vi "String Operations.vi"() -> ()   [LabVIEW 2020]
panel:
  out "offset past replacement":i32
  out "number of replacements":i32
  out "result string 2":string
  in  "Replace str":string
  in  "input str":string="I'm trying to remember something but I couldn't. It's something important , still I forgot. "
  in  "search str":string
  out "result string":string
  out "replaced substring":string
  out "substring":string
  out "len t str":i32
  out "len str3":i32
  out "trimmed string":string
  in  "Str 3":string
  out "concatenated string":string
  in  "Str 2":string
  in  "Str":string
  # "STRING OPERATIONS"
  # "+"
  # "="
  # "t str (2-5)"
  # "string =str3 and substring = str2"
  # "Search and Replace string function"
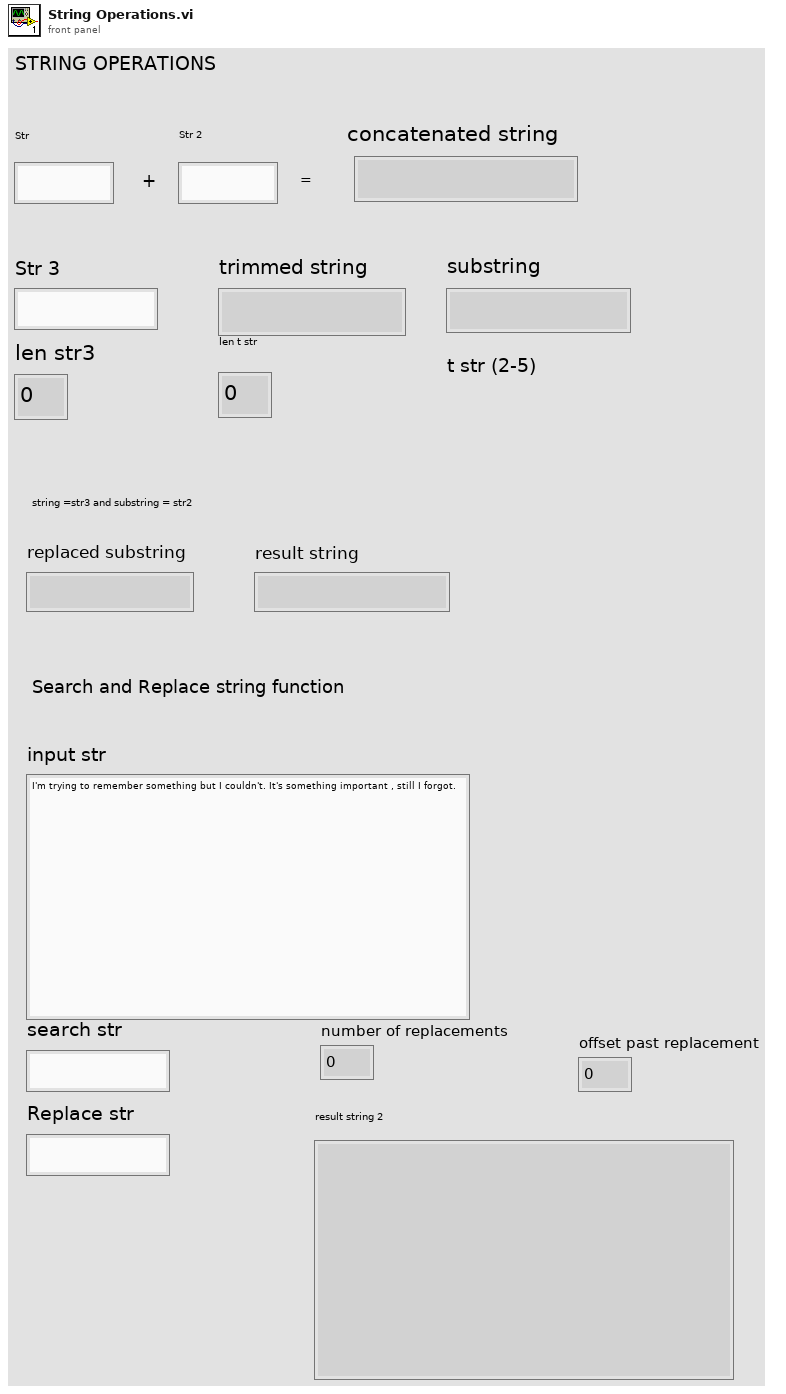
[diagram p1: front panel]
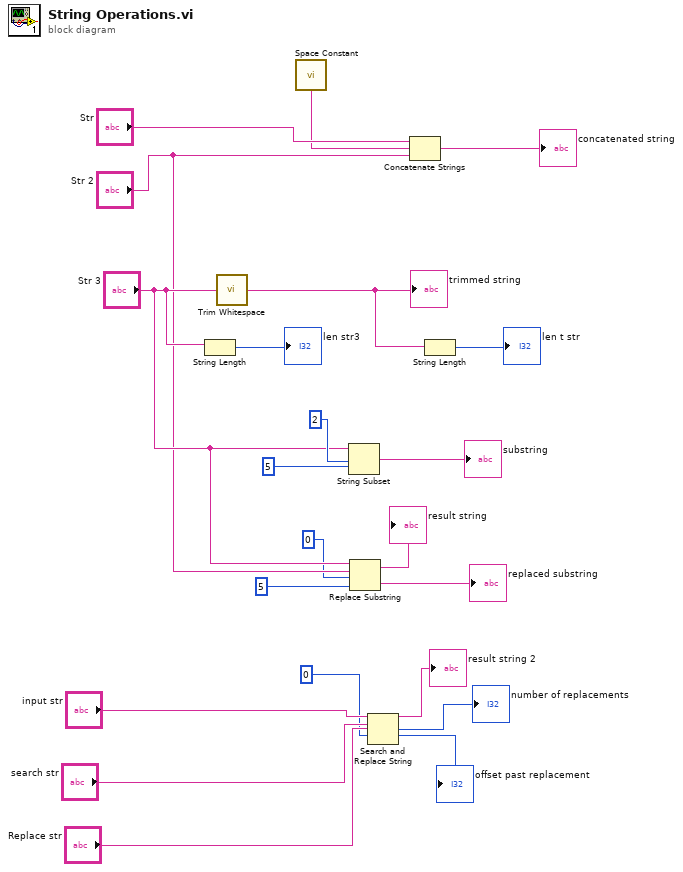
[diagram p0: block diagram]
diagram:
  n1 = String Length(string="Str 3") -> (length=→"len str3":i32)
  n2 = call <vilib>:"Trim Whitespace.vi"("string"="Str 3") -> ("trimmed string"=w17:string)  [unwired: 1 in]
  "trimmed string" <- w17
  n3 = call <vilib>:"Space Constant.vi"() -> ("String"=w20:string)
  n4 = String Subset(string="Str 3", offset (0)=2, length (rest)=5) -> (substring=→"substring":string)
  n5 = Replace Substring(2:5, 3:0, 4:"Str 2", 5:"Str 3") -> (0:→"replaced substring":string, 1:→"result string":string)
  n6 = Search and Replace String(input string="input str", search string="search str", replace string="Replace str", offset=0) -> (result string=→"result string 2":string, number of replacements=→"number of replacements":i32, offset past replacement=→"offset past replacement":i32)  [unwired: 4 in, 1 out]
  n7 = Concatenate Strings("Str", w20, "Str 2") -> (→"concatenated string":string)
  n8 = String Length(string=w17) -> (length=→"len t str":i32)
